vi "read_doubling_spline.vi"(0 "Wavelength":dbl format="%0.2f", 1 "Tuning Spline Path":path, 11 "Error In":errorcluster) -> (3 "BBO Position":i32, 4 "Wavelength Out":dbl format="%0.2f", 15 "Error Out":errorcluster)   [LabVIEW 2023]
uses:
  <vilib>/Utility/file.llb/Read Delimited Spreadsheet (DBL).vi
  <vilib>/Analysis/NI_AALPro.lvlib
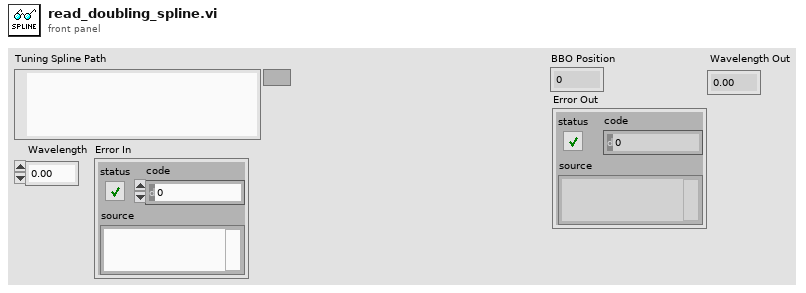
[diagram p1: front panel]
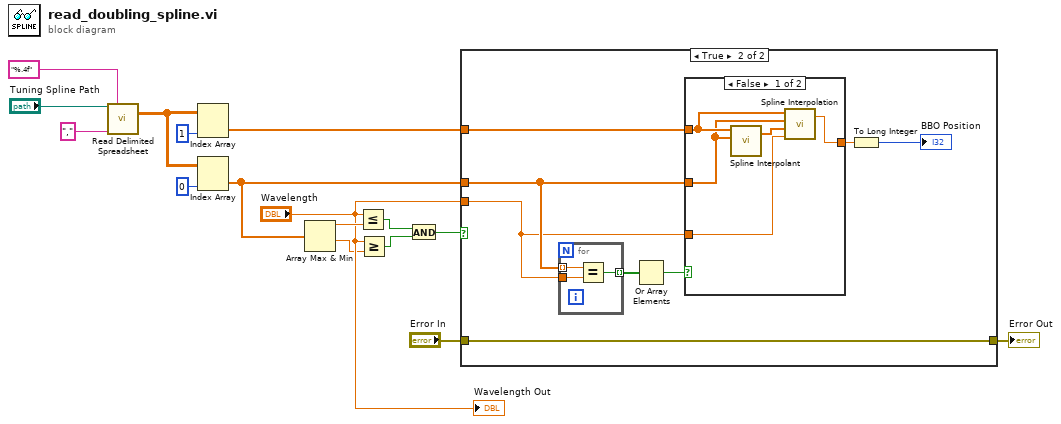
[diagram p0: block diagram]
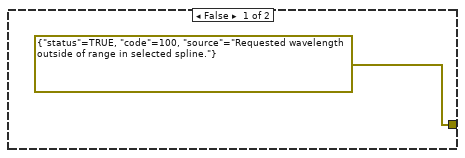
[diagram p2: hidden frame]
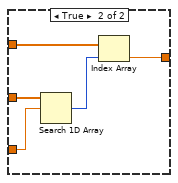
[diagram p3: hidden frame]
diagram:
  n1 = call-poly <vilib>:"Read Delimited Spreadsheet.vi"("file path (dialog if empty)"="Tuning Spline Path", "format (%.3f)"="%.4f", "delimiter (\\t)"="," ("delimiter (\\t)")) -> ("all rows"=w11:dbl[][])  [unwired: 7 in, 5 out]
  n2 = Index Array(array=w11, index (col)=1 ("disabled index (col)")) -> (element=w10:dbl[])  [unwired: 1 in]
  n3 = Index Array(array=w11, index (col)=0 ("disabled index (col)")) -> (element=w9:dbl[])  [unwired: 1 in]
  n4 = Array Max & Min(array=w9) -> (max value=w8:dbl, min value=w6:dbl)  [unwired: 2 out]
  n5 = Less Or Equal?(x="Wavelength", y=w8) -> (x <= y?=w5:bool)
  n6 = Greater Or Equal?(x="Wavelength", y=w6) -> (x >= y?=w4:bool)
  n7 = And(x=w5, y=w4) -> (x .and. y?=w3:bool)
  n8 = case shown="True" w3 {
    tunnel: w9 -> [_ w23]
    tunnel: "Wavelength" -> [_ w22]
    tunnel: w10 -> [_ w21]
    tunnel: "Error In" -> [_ w18]
    tunnel: [errorcluster {"status"=TRUE, "code"=100, "source"="Requested wavelength outside of range in selected spline."} ("Error In") w18] -> w1
    frame False {
    }
    frame True {
      n9 = for {
        tunnel: w23 -> [w38] mode=indexing
        tunnel: w22 -> [w37]
        tunnel: [w36] -> w25 mode=indexing
        n10 = Equal?(x=w38, y=w37) -> (x = y?=w36:bool)
      }
      n11 = Or Array Elements(Boolean array=w25) -> (logical OR=w24:bool)
      n12 = case shown="False" w24 {
        tunnel: w23 -> [w28 w35]
        tunnel: w22 -> [w27 w34]
        tunnel: w21 -> [w29 w33]
        tunnel: [w26 w31] -> w20
        frame False {
          n13 = call <vilib>:"Spline Interpolant.vi"("X"=w28, "Y"=w29) -> ("Interpolant"=w30:dbl[])  [unwired: 2 in, 1 out]
          n14 = call <vilib>:"Spline Interpolation.vi"("x value"=w27, "Interpolant"=w30, "X"=w28, "Y"=w29) -> ("interpolation value"=w26:dbl)  [unwired: 1 out]
        }
        frame True {
          n15 = Search 1D Array(1D array=w35, element=w34) -> (index of element=w32:i32)  [unwired: 1 in]
          n16 = Index Array(array=w33, index=w32) -> (element=w31:dbl)
        }
      }
      n17 = To Long Integer(number=w20) -> (32bit integer=→"BBO Position":i32)
    }
  }
  "Error Out" <- w1
  "Wavelength Out" <- "Wavelength"
